vi "HDI Fiducial Full with Move.vi"(0 "Minimum Match Score":sgl=500.0, 1 "Template File Path":path=path "C:/Users/Admin/Desktop/Main_Module_Assembly/Pattern recognition/templates/color.png", 5 "controller in":refnum<k24>, 11 "error in":errorcluster) -> (4 "Matched?":bool, 6 "Score":dbl, 8 "x rel move":dbl, 10 "y rel move":dbl, 15 "error out":errorcluster)   [LabVIEW 2011]
uses:
  C:/Users/Admin/Desktop/Gantry Code Transfer/source/Code Transfer/Aerotech.A3200.dll
  Aerotech.A3200.dll
  <vilib>/vision/driver/NI_Vision_Acquisition_Software.lvlib
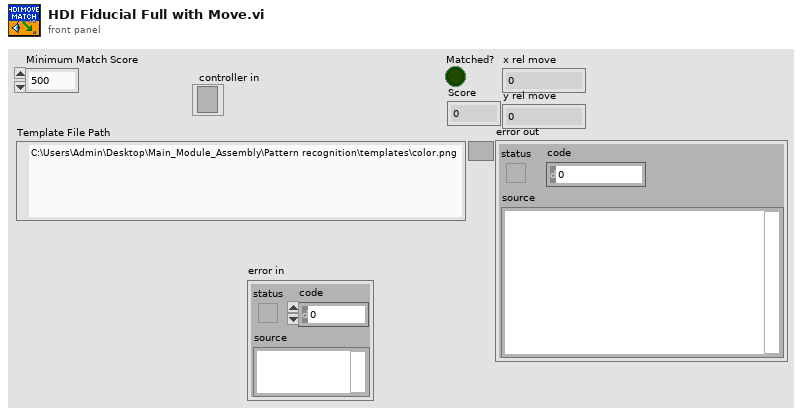
[diagram p1: front panel]
types:
  T1 = typedef "IMAQdx.ctl" = refnum<k21>
  T2 = typedef "IMAQ Image.ctl" = refnum<image>
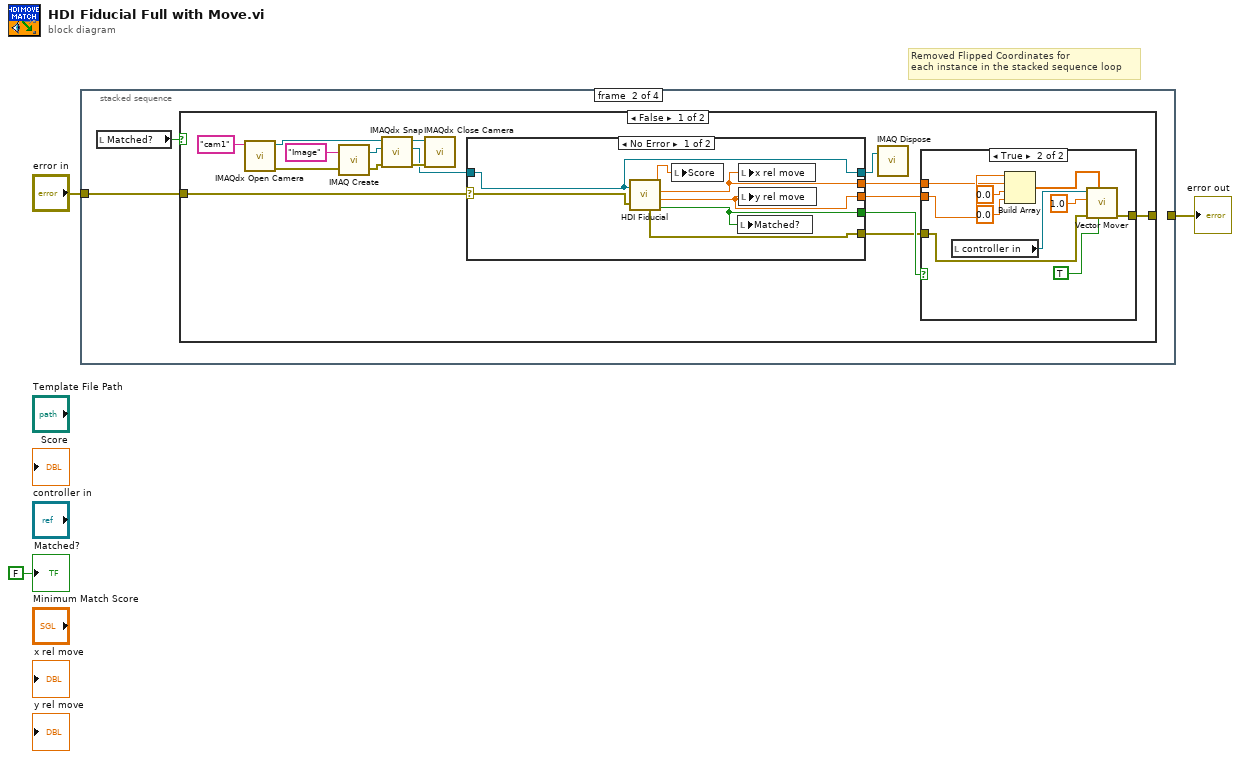
[diagram p0: block diagram]
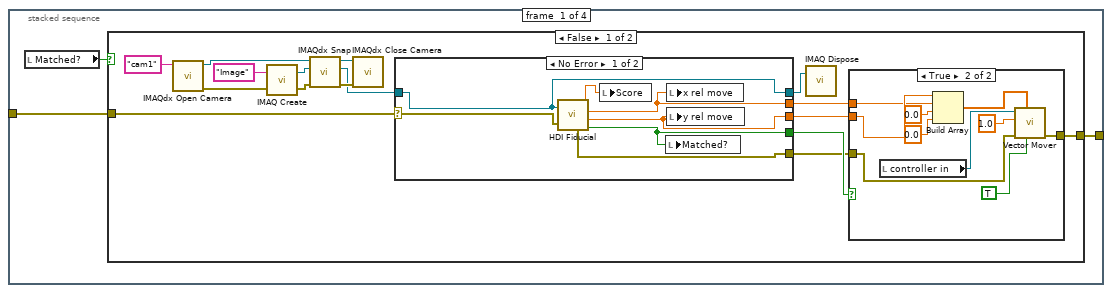
[diagram p2: hidden frame]
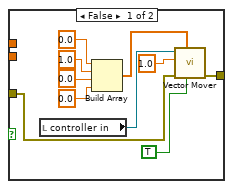
[diagram p3: hidden frame]
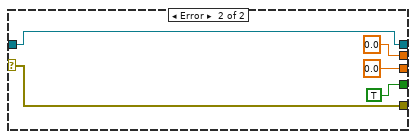
[diagram p4: hidden frame]
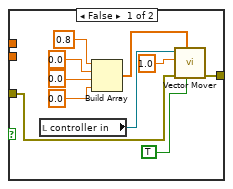
[diagram p6: hidden frame]
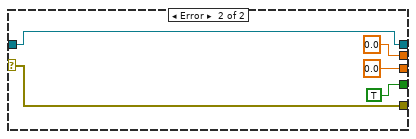
[diagram p7: hidden frame]
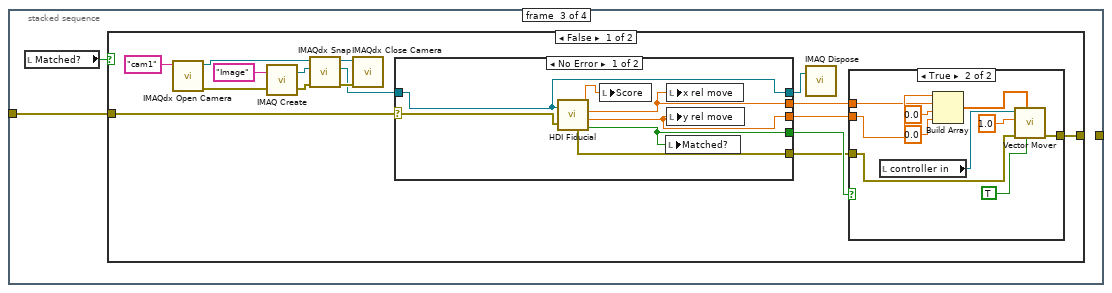
[diagram p9: hidden frame]
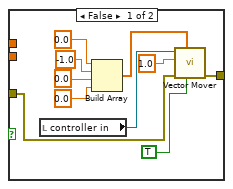
[diagram p10: hidden frame]
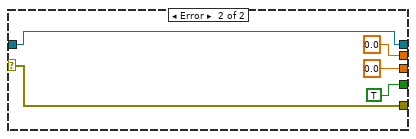
[diagram p11: hidden frame]
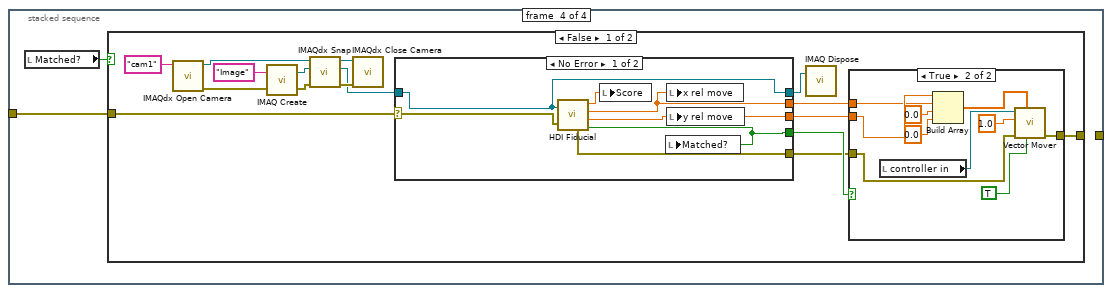
[diagram p13: hidden frame]
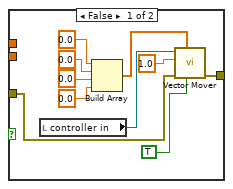
[diagram p14: hidden frame]
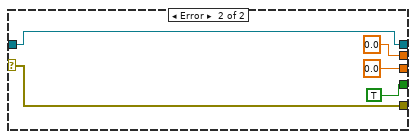
[diagram p15: hidden frame]
diagram:
  # "Removed Flipped Coordinates for \neach instance in the stacked sequence loop"
  n1 = stacked-sequence {
    tunnel: "error in" -> [w6 w57 w108 w159]
    tunnel: [w5 _ _ _] -> w3
    frame #0 {
      n2 = local read "Matched?"() -> (w4:bool)
      n3 = case shown="False" w4 {
        tunnel: w6 -> [w22 w55]
        tunnel: [w19 w55] -> w5
        frame False {
          n4 = call <vilib>:"IMAQdx Open Camera.vi"("Session In"="cam1" ("Interface Name")) -> ("error out"=w13:errorcluster, "Session Out"=w8:T1)  [unwired: 9 in]
          n5 = call "IMAQ Create"("Image Name"="Image", "error in (no error)"=w13) -> ("New Image"=w10:T2, "error out"=w9:errorcluster)  [unwired: 3 in]
          n6 = call <vilib>:"IMAQdx Snap.vi"("error in"=w9, "Image In"=w10, "Session In"=w8) -> ("error out"=w11:errorcluster, "Image Out"=w7:T2, "Session Out"=w12:T1)  [unwired: 6 in]
          n7 = call <vilib>:"IMAQdx Close Camera.vi"("error in"=w11, "Session In"=w12) -> ()  [unwired: 9 in, 1 out]
          n8 = case shown="No Error" w22 {
            selector: w22 -> [w49 w54]
            tunnel: [w43 w54] -> w20
            tunnel: [w45 TRUE ("Matched?")] -> w21
            tunnel: [w47 0.0 ("x rel move")] -> w18
            tunnel: [w46 0.0 ("y rel move")] -> w17
            tunnel: w7 -> [w44 w50]
            tunnel: [w44 w50] -> w16
            frame No Error {
              n9 = call "HDI Fiducial.vi"("error in (no error)"=w49, "Image Src"=w44) -> ("Matched?"=w45:bool, "y rel move"=w46:dbl, "x rel move"=w47:dbl, "Score"=w48:dbl, "error out"=w43:errorcluster)
              n10 = local write "Score"(w48) -> ()
              n11 = local write "Matched?"(w45) -> ()
              n12 = local write "x rel move"(w47) -> ()
              n13 = local write "y rel move"(w46) -> ()
            }
            frame Error {
            }
          }
          n14 = call "IMAQ Dispose"("Image"=w16) -> ()  [unwired: 5 in, 1 out]
          n15 = case shown="True" w21 {
            tunnel: w20 -> [w30 w42]
            tunnel: [w25 w41] -> w19
            tunnel: w18 -> [_ w33]
            tunnel: w17 -> [_ w34]
            frame False {
              n16 = local read "controller in"() -> (w24:refnum<k24>)
              n17 = Build Array(0.0 ("element"), 1.0 ("element"), 0.0 ("element"), 0.0 ("element")) -> (w27:dbl[])
              n18 = call "Vector Mover.vi"("Absolute/Relative (F/T)"=TRUE, "Movement Vector"=w27, "error in (no error)"=w30, "Vector Speed"=1.0, "controller in"=w24) -> ("error out"=w25:errorcluster)  [unwired: 1 in, 3 out]
            }
            frame True {
              n19 = local read "controller in"() -> (w35:refnum<k24>)
              n20 = Build Array(w34, w33, 0.0 ("element"), 0.0 ("element")) -> (w36:dbl[])
              n21 = call "Vector Mover.vi"("Absolute/Relative (F/T)"=TRUE, "Movement Vector"=w36, "error in (no error)"=w42, "Vector Speed"=1.0, "controller in"=w35) -> ("error out"=w41:errorcluster)  [unwired: 1 in, 3 out]
            }
          }
        }
        frame True {
        }
      }
    }
    frame #1 {
      n22 = local read "Matched?"() -> (w56:bool)
      n23 = case shown="False" w56 {
        tunnel: w57 -> [w73 w106]
        tunnel: [w70 w106] -> _
        frame False {
          n24 = call <vilib>:"IMAQdx Open Camera.vi"("Session In"="cam1" ("Interface Name")) -> ("error out"=w64:errorcluster, "Session Out"=w59:T1)  [unwired: 9 in]
          n25 = call "IMAQ Create"("Image Name"="Image", "error in (no error)"=w64) -> ("New Image"=w61:T2, "error out"=w60:errorcluster)  [unwired: 3 in]
          n26 = call <vilib>:"IMAQdx Snap.vi"("error in"=w60, "Image In"=w61, "Session In"=w59) -> ("error out"=w62:errorcluster, "Image Out"=w58:T2, "Session Out"=w63:T1)  [unwired: 6 in]
          n27 = call <vilib>:"IMAQdx Close Camera.vi"("error in"=w62, "Session In"=w63) -> ()  [unwired: 9 in, 1 out]
          n28 = case shown="No Error" w73 {
            selector: w73 -> [w100 w105]
            tunnel: [w94 w105] -> w71
            tunnel: [w96 TRUE ("Matched?")] -> w72
            tunnel: [w98 0.0 ("x rel move")] -> w69
            tunnel: [w97 0.0 ("y rel move")] -> w68
            tunnel: w58 -> [w95 w101]
            tunnel: [w95 w101] -> w67
            frame No Error {
              n29 = call "HDI Fiducial.vi"("error in (no error)"=w100, "Image Src"=w95) -> ("Matched?"=w96:bool, "y rel move"=w97:dbl, "x rel move"=w98:dbl, "Score"=w99:dbl, "error out"=w94:errorcluster)
              n30 = local write "Score"(w99) -> ()
              n31 = local write "Matched?"(w96) -> ()
              n32 = local write "x rel move"(w98) -> ()
              n33 = local write "y rel move"(w97) -> ()
            }
            frame Error {
            }
          }
          n34 = call "IMAQ Dispose"("Image"=w67) -> ()  [unwired: 5 in, 1 out]
          n35 = case shown="True" w72 {
            tunnel: w71 -> [w81 w93]
            tunnel: [w75 w92] -> w70
            tunnel: w69 -> [_ w84]
            tunnel: w68 -> [_ w85]
            frame False {
              n36 = local read "controller in"() -> (w74:refnum<k24>)
              n37 = Build Array(0.8 ("element"), 0.0 ("element"), 0.0 ("element"), 0.0 ("element")) -> (w78:dbl[])
              n38 = call "Vector Mover.vi"("Absolute/Relative (F/T)"=TRUE, "Movement Vector"=w78, "error in (no error)"=w81, "Vector Speed"=1.0, "controller in"=w74) -> ("error out"=w75:errorcluster)  [unwired: 1 in, 3 out]
            }
            frame True {
              n39 = local read "controller in"() -> (w87:refnum<k24>)
              n40 = Build Array(w85, w84, 0.0 ("element"), 0.0 ("element")) -> (w86:dbl[])
              n41 = call "Vector Mover.vi"("Absolute/Relative (F/T)"=TRUE, "Movement Vector"=w86, "error in (no error)"=w93, "Vector Speed"=1.0, "controller in"=w87) -> ("error out"=w92:errorcluster)  [unwired: 1 in, 3 out]
            }
          }
        }
        frame True {
        }
      }
    }
    frame #2 {
      n42 = local read "Matched?"() -> (w107:bool)
      n43 = case shown="False" w107 {
        tunnel: w108 -> [w124 w157]
        tunnel: [w121 w157] -> _
        frame False {
          n44 = call <vilib>:"IMAQdx Open Camera.vi"("Session In"="cam1" ("Interface Name")) -> ("error out"=w115:errorcluster, "Session Out"=w110:T1)  [unwired: 9 in]
          n45 = call "IMAQ Create"("Image Name"="Image", "error in (no error)"=w115) -> ("New Image"=w112:T2, "error out"=w111:errorcluster)  [unwired: 3 in]
          n46 = call <vilib>:"IMAQdx Snap.vi"("error in"=w111, "Image In"=w112, "Session In"=w110) -> ("error out"=w113:errorcluster, "Image Out"=w109:T2, "Session Out"=w114:T1)  [unwired: 6 in]
          n47 = call <vilib>:"IMAQdx Close Camera.vi"("error in"=w113, "Session In"=w114) -> ()  [unwired: 9 in, 1 out]
          n48 = case shown="No Error" w124 {
            selector: w124 -> [w151 w156]
            tunnel: [w145 w156] -> w122
            tunnel: [w147 TRUE ("Matched?")] -> w123
            tunnel: [w149 0.0 ("x rel move")] -> w120
            tunnel: [w148 0.0 ("y rel move")] -> w119
            tunnel: w109 -> [w146 w152]
            tunnel: [w146 w152] -> w118
            frame No Error {
              n49 = call "HDI Fiducial.vi"("error in (no error)"=w151, "Image Src"=w146) -> ("Matched?"=w147:bool, "y rel move"=w148:dbl, "x rel move"=w149:dbl, "Score"=w150:dbl, "error out"=w145:errorcluster)
              n50 = local write "Score"(w150) -> ()
              n51 = local write "Matched?"(w147) -> ()
              n52 = local write "x rel move"(w149) -> ()
              n53 = local write "y rel move"(w148) -> ()
            }
            frame Error {
            }
          }
          n54 = call "IMAQ Dispose"("Image"=w118) -> ()  [unwired: 5 in, 1 out]
          n55 = case shown="True" w123 {
            tunnel: w122 -> [w132 w144]
            tunnel: [w126 w143] -> w121
            tunnel: w120 -> [_ w135]
            tunnel: w119 -> [_ w136]
            frame False {
              n56 = local read "controller in"() -> (w125:refnum<k24>)
              n57 = Build Array(0.0 ("element"), -1.0 ("element"), 0.0 ("element"), 0.0 ("element")) -> (w129:dbl[])
              n58 = call "Vector Mover.vi"("Absolute/Relative (F/T)"=TRUE, "Movement Vector"=w129, "error in (no error)"=w132, "Vector Speed"=1.0, "controller in"=w125) -> ("error out"=w126:errorcluster)  [unwired: 1 in, 3 out]
            }
            frame True {
              n59 = local read "controller in"() -> (w137:refnum<k24>)
              n60 = Build Array(w136, w135, 0.0 ("element"), 0.0 ("element")) -> (w138:dbl[])
              n61 = call "Vector Mover.vi"("Absolute/Relative (F/T)"=TRUE, "Movement Vector"=w138, "error in (no error)"=w144, "Vector Speed"=1.0, "controller in"=w137) -> ("error out"=w143:errorcluster)  [unwired: 1 in, 3 out]
            }
          }
        }
        frame True {
        }
      }
    }
    frame #3 {
      n62 = local read "Matched?"() -> (w158:bool)
      n63 = case shown="False" w158 {
        tunnel: w159 -> [w175 w208]
        tunnel: [w172 w208] -> _
        frame False {
          n64 = call <vilib>:"IMAQdx Open Camera.vi"("Session In"="cam1" ("Interface Name")) -> ("error out"=w166:errorcluster, "Session Out"=w161:T1)  [unwired: 9 in]
          n65 = call "IMAQ Create"("Image Name"="Image", "error in (no error)"=w166) -> ("New Image"=w163:T2, "error out"=w162:errorcluster)  [unwired: 3 in]
          n66 = call <vilib>:"IMAQdx Snap.vi"("error in"=w162, "Image In"=w163, "Session In"=w161) -> ("error out"=w164:errorcluster, "Image Out"=w160:T2, "Session Out"=w165:T1)  [unwired: 6 in]
          n67 = call <vilib>:"IMAQdx Close Camera.vi"("error in"=w164, "Session In"=w165) -> ()  [unwired: 9 in, 1 out]
          n68 = case shown="No Error" w175 {
            selector: w175 -> [w202 w207]
            tunnel: [w197 w207] -> w173
            tunnel: [w196 TRUE ("Matched?")] -> w174
            tunnel: [w200 0.0 ("x rel move")] -> w171
            tunnel: [w198 0.0 ("y rel move")] -> w170
            tunnel: w160 -> [w201 w204]
            tunnel: [w201 w204] -> w169
            frame No Error {
              n69 = call "HDI Fiducial.vi"("error in (no error)"=w202, "Image Src"=w201) -> ("Matched?"=w196:bool, "y rel move"=w198:dbl, "x rel move"=w200:dbl, "Score"=w199:dbl, "error out"=w197:errorcluster)
              n70 = local write "Score"(w199) -> ()
              n71 = local write "Matched?"(w196) -> ()
              n72 = local write "x rel move"(w200) -> ()
              n73 = local write "y rel move"(w198) -> ()
            }
            frame Error {
            }
          }
          n74 = call "IMAQ Dispose"("Image"=w169) -> ()  [unwired: 5 in, 1 out]
          n75 = case shown="True" w174 {
            tunnel: w173 -> [w183 w195]
            tunnel: [w177 w194] -> w172
            tunnel: w171 -> [_ w186]
            tunnel: w170 -> [_ w187]
            frame False {
              n76 = local read "controller in"() -> (w176:refnum<k24>)
              n77 = Build Array(0.0 ("element"), 0.0 ("element"), 0.0 ("element"), 0.0 ("element")) -> (w180:dbl[])
              n78 = call "Vector Mover.vi"("Absolute/Relative (F/T)"=TRUE, "Movement Vector"=w180, "error in (no error)"=w183, "Vector Speed"=1.0, "controller in"=w176) -> ("error out"=w177:errorcluster)  [unwired: 1 in, 3 out]
            }
            frame True {
              n79 = local read "controller in"() -> (w188:refnum<k24>)
              n80 = Build Array(w187, w186, 0.0 ("element"), 0.0 ("element")) -> (w189:dbl[])
              n81 = call "Vector Mover.vi"("Absolute/Relative (F/T)"=TRUE, "Movement Vector"=w189, "error in (no error)"=w195, "Vector Speed"=1.0, "controller in"=w188) -> ("error out"=w194:errorcluster)  [unwired: 1 in, 3 out]
            }
          }
        }
        frame True {
        }
      }
    }
  }
  "error out" <- w3
  "Matched?" <- FALSE ("Matched?")
